vi "pane_origin.vi"   [LabVIEW 2025]
doc: "This VI is used for demonstrating the value setting of the pane origin of the front panel.\n\nMichael Panganiban\nSr. Hardware Test Engineer\nFresh Consulting, Inc."
uses:
  <vilib>/Utility/miscctls.llb/LVPointTypeDef.ctl
panel:
  # "Pane Origin"
types:
  T1 = typedef "LVPointTypeDef.ctl" = cluster{"Horizontal":i16, "Vertical":i16}
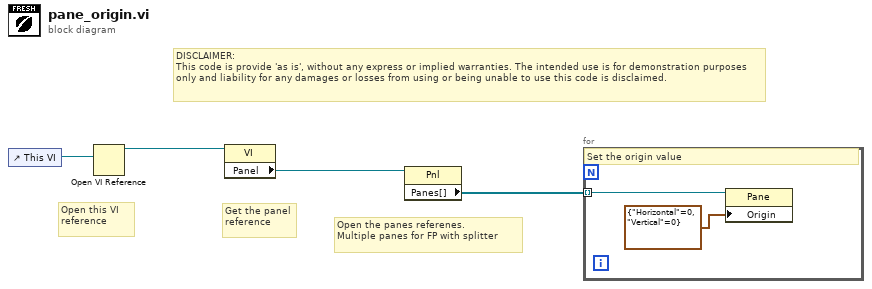
[diagram p0: block diagram]
diagram:
  # "DISCLAIMER:\nThis code is provide 'as is', without any express or implied warranties. The intended use is for demonstration purposes only and liability for any damages or losses from using or being unable to use this code is disclaimed."
  # "Open the panes referenes.\nMultiple panes for FP with splitter"
  # "Get the panel reference"
  # "Open this VI reference"
  n1 = control-ref of="This VI"() -> (w4:refnum<vi>)
  n2 = Open VI Reference(vi path=w4) -> (vi reference=w3:refnum<vi>)  [unwired: 5 in, 1 out]
  n3 = property class="VI"(reference=w3) -> ("Panel"=w2:refnum<vi>)  [unwired: 1 in, 2 out]
  n4 = property class="Pnl"(reference=w2) -> ("Panes[]"=w1:refnum<vi>[])  [unwired: 1 in, 2 out]
  n5 = for {
    tunnel: w1 -> [w6] mode=indexing
    # "Set the origin value"
    n6 = property class="Pane"(reference=w6, "Origin"=T1 {"Horizontal"=0, "Vertical"=0}) -> ()  [unwired: 1 in, 2 out]
  }
